vi "FIFO Clear All.vi"(8 "error in (no error)":errorcluster, 11 "Csatorna jellemzõk":T1[](array[typedef])) -> (0 "error out":errorcluster, 3 "Csatorna jellemzõk 2":T1[](array[typedef]))   [LabVIEW 2014]
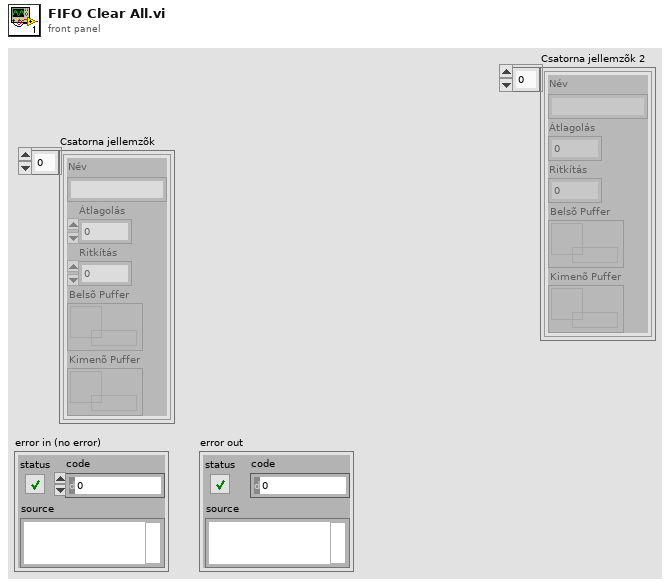
[diagram p1: front panel]
types:
  T1 = typedef "Csatorna jellemzõk.ctl" = cluster{"Név":string, "Átlagolás":i32, "Ritkítás":i32, "Belsõ Puffer":refnum<queue>, "Kimenõ Puffer":refnum<queue>}
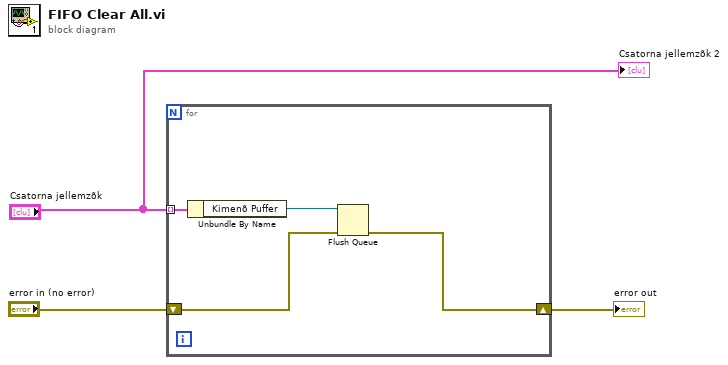
[diagram p0: block diagram]
diagram:
  n1 = for {
    tunnel: "Csatorna jellemzõk" -> [w7] mode=indexing
    shift-right: [w4] -> w3
    shift-left: "error in (no error)" -> [w5]
    n2 = Unbundle By Name(w7) -> ("Kimenõ Puffer"=w6:refnum<queue>)
    n3 = Flush Queue(queue=w6, error in (no error)=w5) -> (error out=w4:errorcluster)  [unwired: 2 out]
  }
  "error out" <- w3
  "Csatorna jellemzõk 2" <- "Csatorna jellemzõk"
